vi "DataGraph_Calc_Rectangle_Y.vi"(4 "X Maximum Index":u32, 5 "X Minimum Index":u32, 7 "Y Minimum":dbl, 8 "Y Maximum":dbl, 9 "Raw Y Array":dbl[](array[numeric])) -> (3 "Allow Index Bool":bool[](array[boolean]))   [LabVIEW 2018, in "DataGraphXControl.xctl"]
uses:
  DataGraphXControl.xctl
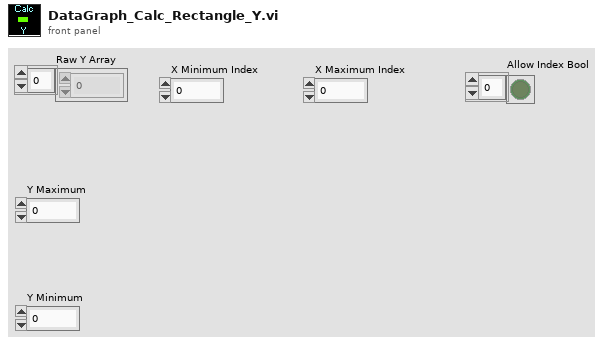
[diagram p1: front panel]
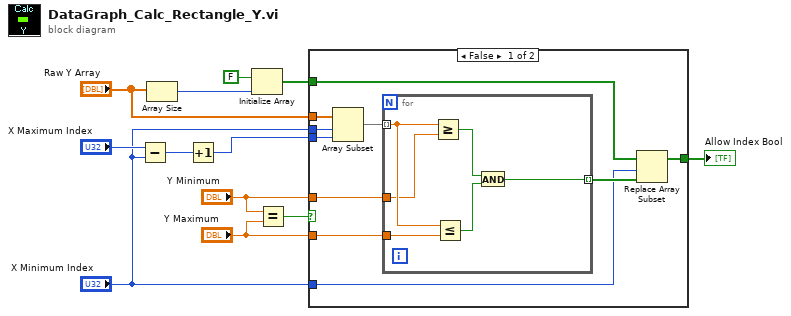
[diagram p0: block diagram]
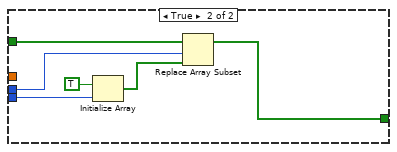
[diagram p2: hidden frame]
diagram:
  n1 = Subtract(x="X Maximum Index", y="X Minimum Index") -> (x-y=w9:u32)
  n2 = Array Size(array="Raw Y Array") -> (size(s)=w11:i32)
  n3 = Increment(x=w9) -> (x+1=w1:u32)
  n4 = Initialize Array(FALSE, w11) -> (w8:bool[])
  n5 = Equal?(x="Y Minimum", y="Y Maximum") -> (x = y?=w4:bool)
  n6 = case shown="False" w4 {
    tunnel: w8 -> [w21 w34]
    tunnel: "X Minimum Index" -> [w20 _]
    tunnel: [w19 w29] -> w7
    tunnel: "Y Minimum" -> [w18 _]
    tunnel: "Y Maximum" -> [w17 _]
    tunnel: "Raw Y Array" -> [w16 _]
    tunnel: "X Minimum Index" -> [w15 w33]
    tunnel: w1 -> [w14 w31]
    frame False {
      n7 = Array Subset(array=w16, index=w15, length=w14) -> (w13:dbl[])
      n8 = for {
        tunnel: w13 -> [w28] mode=indexing
        tunnel: [w25] -> w22 mode=indexing
        tunnel: w18 -> [w24]
        tunnel: w17 -> [w23]
        n9 = Greater Or Equal?(x=w28, y=w24) -> (x >= y?=w27:bool)
        n10 = Less Or Equal?(x=w28, y=w23) -> (x <= y?=w26:bool)
        n11 = And(x=w27, y=w26) -> (x .and. y?=w25:bool)
      }
      n12 = Replace Array Subset(array=w21, new element=w22, index=w20) -> (w19:bool[])
    }
    frame True {
      n13 = Initialize Array(TRUE, w31) -> (w30:bool[])
      n14 = Replace Array Subset(array=w34, new element=w30, index=w33) -> (w29:bool[])
    }
  }
  "Allow Index Bool" <- w7
